vi "Read View Channel info.vi"(8 "error in":errorcluster, 11 "channel in":refnum<class "Cfg Channel.lvclass">) -> (0 "error out":errorcluster, 2 "channel info":T1, 3 "channel out":refnum<class "Cfg Channel.lvclass">)   [LabVIEW 2013, in "Cfg Channel.lvclass"]
uses:
  Cfg Channel.lvclass
  ChannelDisplayInfo.ctl
  Cfg Channel.lvclass/Cfg Channel.ctl
  chcfg/channel config object.lvclass/channel config object.ctl
  chcfg/Read IO.vi
  chcfg/Read sensor ID.vi
  chcfg/Read channel name.vi
  chcfg/Read description.vi
  chcfg/channel config object.lvclass
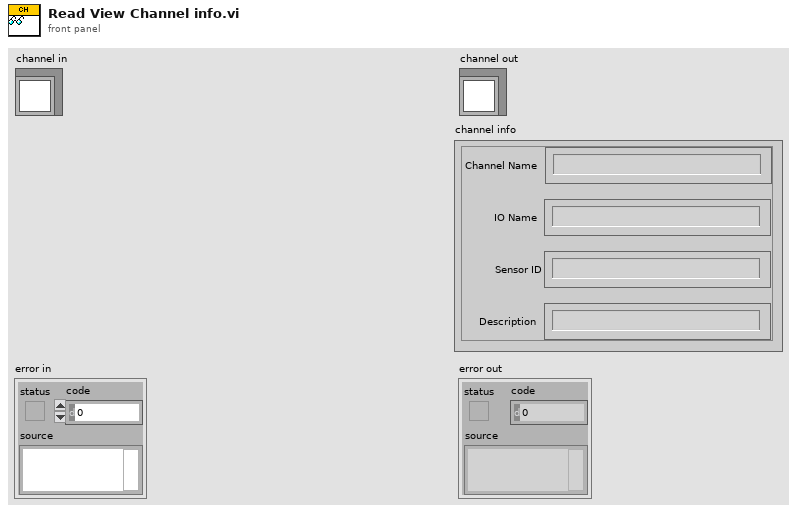
[diagram p1: front panel]
types:
  T1 = typedef "Cfg Channel.lvclass/ChannelDisplayInfo.ctl" = cluster{"IO Name":string, "Sensor ID":string, "Channel Name":string, "Description ":string}
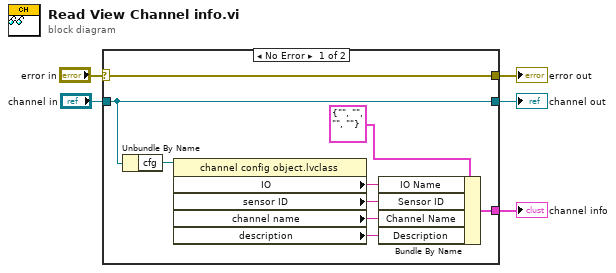
[diagram p0: block diagram]
diagram:
  n1 = case shown="No Error" "error in" {
    selector: "error in" -> [w14 w15]
    tunnel: [w14 w15] -> w4
    tunnel: [w13 w16] -> w2
    tunnel: "channel in" -> [w13 w16]
    tunnel: [w12 _] -> w1
    frame No Error {
      n2 = Unbundle By Name(w13) -> ("cfg"=w10:refnum<class "channel config object.lvclass">)
      n3 = property class="channel config object.lvclass"(reference=w10) -> ("IO "=w9:string, "sensor ID"=w8:string, "channel name"=w7:string, "description"=w6:string)  [unwired: 1 in, 2 out]
      n4 = Bundle By Name(cluster=T1 {"IO Name"="", "Sensor ID"="", "Channel Name"="", "Description "=""} ("channel info"), "IO Name"=w9, "Sensor ID"=w8, "Channel Name"=w7, "Description"=w6) -> (w12:T1)
    }
    frame Error {
    }
  }
  "error out" <- w4
  "channel out" <- w2
  "channel info" <- w1
